vi "New-View.vi"(8 "error in (no error)":errorcluster) -> (0 "error out":errorcluster, 3 "View out":refnum<class "View.lvclass">)   [LabVIEW 2020, in "GLF.lvlib" / "View.lvclass"]
uses:
  View.lvclass
  View.lvclass/View.ctl
  DVR--cluster.ctl
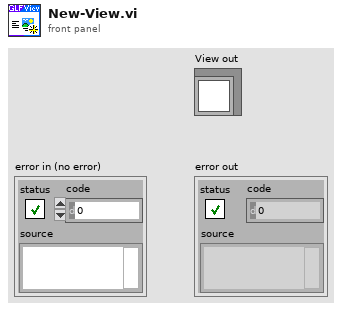
[diagram p1: front panel]
types:
  T1 = typedef "GLF.lvlib/View.lvclass/DVR--cluster.ctl" = cluster{"foo":dbl}
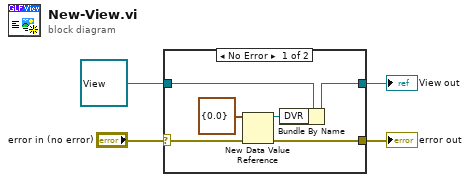
[diagram p0: block diagram]
diagram:
  n1 = case shown="No Error" "error in (no error)" {
    selector: "error in (no error)" -> [w8 w12]
    tunnel: [w5 w12] -> w3
    tunnel: [w6 w11] -> w1
    tunnel: refnum<class "View.lvclass"> refnum ("View in") -> [w7 w11]
    frame No Error {
      n2 = New Data Value Reference(data value=T1 {"foo"=0.0} ("DVR"), error in=w8) -> (data value reference=w9:refnum<data-value>, error out=w5:errorcluster)
      n3 = Bundle By Name(cluster=w7, "DVR"=w9) -> (w6:refnum<class "View.lvclass">)
    }
    frame Error {
    }
  }
  "error out" <- w3
  "View out" <- w1
